vi "Remove.vi"(8 "error in":errorcluster, 11 "Module ID":i32=-1) -> (0 "error out":errorcluster, 2 "empty":bool)   [LabVIEW 2020, in "NI DAQ Aug 25.lvlib" / "Clone Registration.lvlib"]
doc: "Remove the specified cloneable module ID from the registry.\n_____\nBased on DQMH Dev Tools: Project Template 7.1.0.1499."
uses:
  Clone Registration.lvlib
  Action--enum.ctl
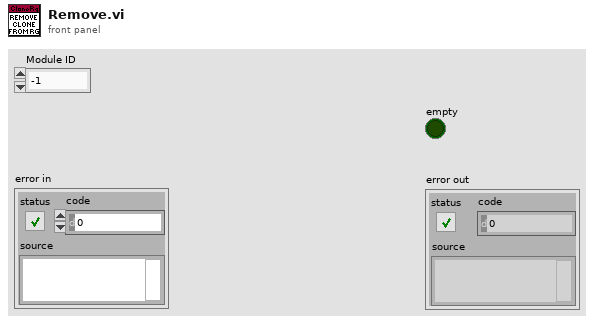
[diagram p1: front panel]
types:
  T1 = typedef "NI DAQ Aug 25.lvlib/Clone Registration.lvlib/Action--enum.ctl" = enum16{"Init", "Add Instance", "Remove Instance", "List Instances", "Is First?"}
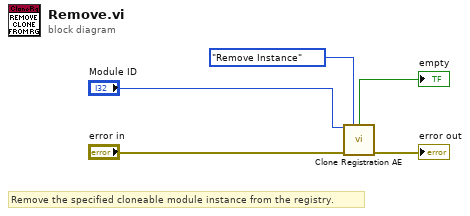
[diagram p0: block diagram]
diagram:
  # "Remove the specified cloneable module instance from the registry."
  n1 = call "Clone Registration AE.vi"("Module ID"="Module ID", "Action"=Action--enum."Remove Instance", "error in"="error in") -> ("empty"=→"empty":bool, "error out"=→"error out":errorcluster)  [unwired: 4 in, 7 out]
